vi "Group1Assignment1.vi"() -> ()   [LabVIEW 2020]
doc: "This example performs a serial port write and a serial port read. The parameters set for the serial port must match the parameters of the connected instrument or device. The VISA Configure Serial Port VI sets the configuration parameters. The front panel displays the controls used to configure the basic parameters, such as baud rate, data bits, and parity. The VI passes the VISA resource name to other VIs that perform operations on that VISA resource. The VISA Write function sends a command to the serial device and the VISA Read function returns data based on the command. The VISA Close function then closes the reference to the serial device. It is important to close the reference; otherwise, further communication through that port might not be possible."
uses:
  <vilib>/Utility/file.llb/Write Delimited Spreadsheet (string).vi
  <vilib>/Instr/_visa.llb/VISA Configure Serial Port (Instr).vi
  <vilib>/Utility/file.llb/Read Delimited Spreadsheet (string).vi
  d40ec6dd-3ecf-4240-bb8a-4498ac5227aa.vi
panel:
  out "Table Control":string[][](table)
  out "2D Picture":picture
  in  "error in (no error)":errorcluster
  out "?":u32
  out "Response":string
  in  "VISA resource name":refnum<visa-resource-name>="COM1"
  # "Overview: Demonstrates the use of the VISA functions to send a single command to a serial instrument and read a response.\nRequirements: NI-VISA Driver\nInstructions:\n1. Ensure the resource specified by the VISA resource name is a valid serial device.\n2. Run the VI.\n3. If your instrument recognizes the \"*IDN?\" command, it should return a Response."
  # "Note: For an example of how to perform continuous serial communication in a loop, open the Continuous Serial Write and Read.vi in the same folder as this example."
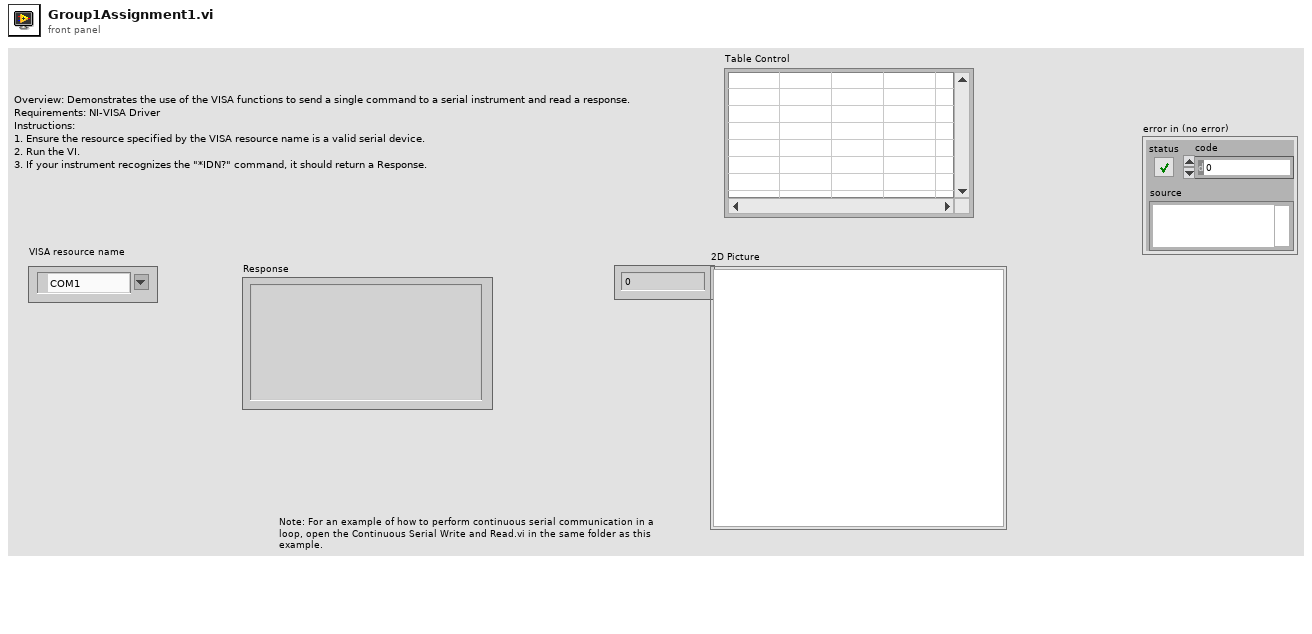
[diagram p1: front panel]
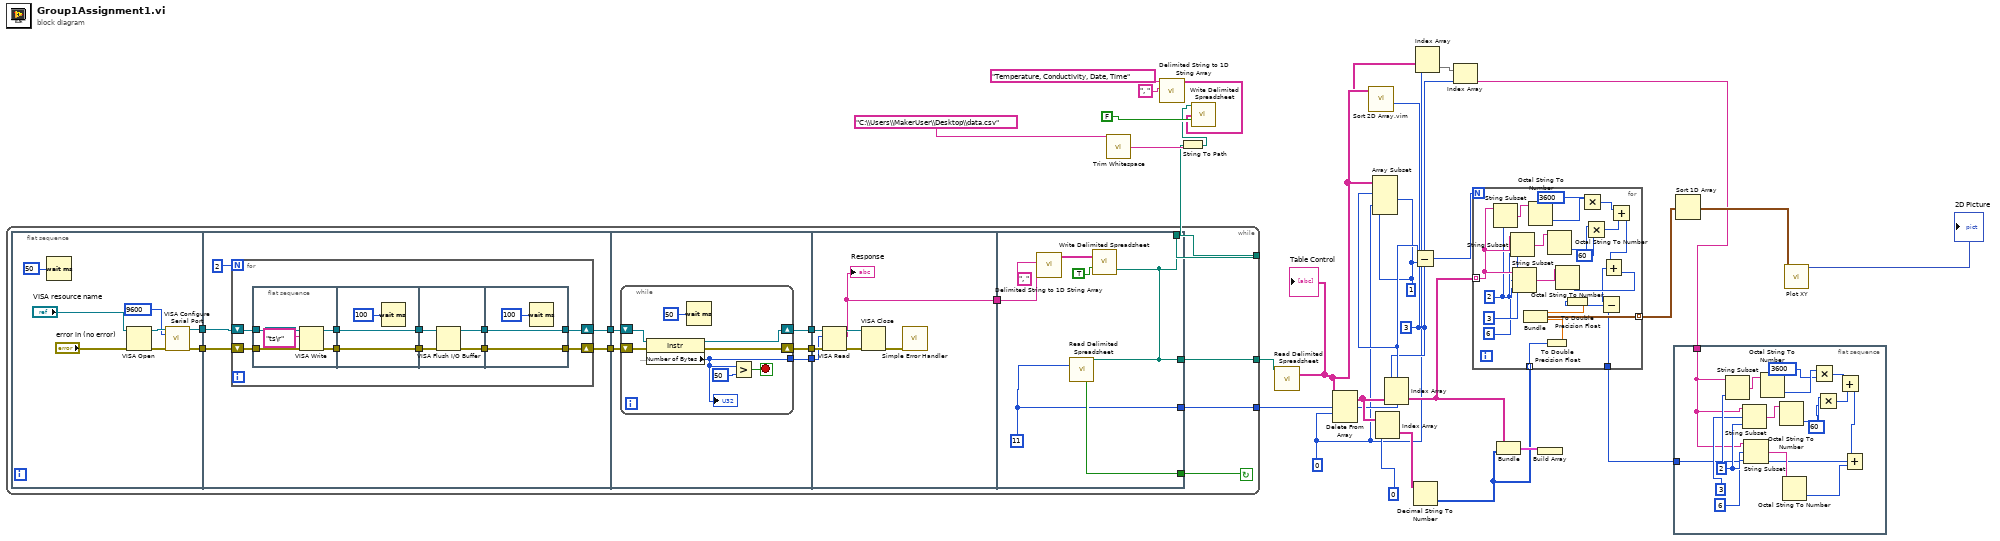
[diagram p0: block diagram]
diagram:
  w5 = 1
  w2 = 3
  w1 = 0
  n1 = call <vilib>:"Trim Whitespace.vi"("string"="C:\\Users\\MakerUser\\Desktop\\data.csv") -> ("trimmed string"=w26:string)  [unwired: 1 in]
  n2 = call <vilib>:"Delimited String to 1D String Array.vi"("delimiter"=", ", "delimited string"="Temperature, Conductivity, Date, Time") -> ("string array"=w23:string[])  [unwired: 9 in]
  n3 = String To Path(string=w26) -> (path=w20:path)
  n4 = while {
    tunnel: w20 -> [w31]
    tunnel: [w29] -> w19
    tunnel: [w28] -> w6
    stop <- w30 continue-if-true
    n5 = flat-sequence {
      tunnel: [w41] -> w39
      tunnel: [w40] -> w38
      tunnel: w39 -> [w52]
      tunnel: w38 -> [w51]
      tunnel: [w49] -> w37
      tunnel: [w48] -> w36
      tunnel: w37 -> [w82]
      tunnel: w36 -> [w81]
      tunnel: [w80] -> w35
      tunnel: [w79] -> w34
      tunnel: [w78] -> w33
      tunnel: w35 -> [w97]
      tunnel: w34 -> [w96]
      tunnel: w33 -> [w95]
      tunnel: [w91] -> w32
      tunnel: w32 -> [w104]
      tunnel: w31 -> [w99]
      tunnel: [w100] -> w30
      tunnel: [w99] -> w29
      tunnel: [w98] -> w28
      frame #0 {
        n6 = Wait (ms)(milliseconds to wait=50) -> ()  [unwired: 1 out]
        n7 = VISA Open(error in (no error)="error in (no error)", VISA resource name="VISA resource name") -> (VISA resource name=w45:refnum<visa-resource-name>, error out=w44:errorcluster)  [unwired: 3 in]
        n8 = call-poly "VISA Configure Serial Port"("VISA resource name"=w45, "baud rate (9600)"=u32 9600, "error in (no error)"=w44) -> ("VISA resource name out"=w41:refnum<visa-resource-name>, "error out"=w40:errorcluster)  [unwired: 6 in, 5 out]
      }
      frame #1 {
        n9 = for {
          N: 2 -> [_]
          shift-right: [w55] -> w49
          shift-left: w52 -> [w54]
          shift-right: [w56] -> w48
          shift-left: w51 -> [w53]
          n10 = flat-sequence {
            tunnel: w54 -> [w66]
            tunnel: w53 -> [w65]
            tunnel: [w64] -> w62
            tunnel: [w63] -> w59
            tunnel: w62 -> [w70]
            tunnel: [w70] -> w61
            tunnel: [w69] -> w60
            tunnel: w59 -> [w69]
            tunnel: w61 -> [w74]
            tunnel: w60 -> [w73]
            tunnel: [w72] -> w58
            tunnel: [w71] -> w57
            tunnel: [w77] -> w55
            tunnel: w58 -> [w77]
            tunnel: [w76] -> w56
            tunnel: w57 -> [w76]
            frame #0 {
              n11 = VISA Write(VISA resource name=w66, write buffer="ts\r", error in (no error)=w65) -> (VISA resource name out=w63:refnum<visa-resource-name>, error out=w64:errorcluster)  [unwired: 1 out]
            }
            frame #1 {
              n12 = Wait (ms)(milliseconds to wait=u32 100) -> ()  [unwired: 1 out]
            }
            frame #2 {
              n13 = VISA Flush I/O Buffer(VISA resource name=w73, error in (no error)=w74) -> (VISA resource name out=w72:refnum<visa-resource-name>, error out=w71:errorcluster)  [unwired: 1 in]
            }
            frame #3 {
              n14 = Wait (ms)(milliseconds to wait=u32 100) -> ()  [unwired: 1 out]
            }
          }
        }
      }
      frame #2 {
        n15 = while {
          tunnel: [w85] -> w78
          shift-right: [w88] -> w79
          shift-left: w81 -> [w83]
          shift-right: [w89] -> w80
          shift-left: w82 -> [w84]
          stop <- w86 stop-if-true
          n16 = property class="Instr"(reference=w84, error in=w83) -> (reference out=w89:refnum<visa-resource-name>, error out=w88:errorcluster, "Serial Settings:Number of Bytes at Serial Port"=w85:u32)
          "?" <- w85
          n17 = Wait (ms)(milliseconds to wait=50) -> ()  [unwired: 1 out]
          n18 = Greater?(x=w85, y=u32 50 ("Serial Settings:Number of Bytes at Serial Port")) -> (0:w86:bool)
        }
      }
      frame #3 {
        n19 = VISA Read(VISA resource name=w97, byte count=w95, error in (no error)=w96) -> (VISA resource name out=w93:refnum<visa-resource-name>, read buffer=w91:string, error out=w92:errorcluster)  [unwired: 1 out]
        "Response" <- w91
        n20 = VISA Close(VISA resource name=w93, error in (no error)=w92) -> (error out=w94:errorcluster)
        n21 = call <vilib>:"Simple Error Handler.vi"("error in (no error)"=w94) -> ()  [unwired: 1 in, 8 out]
      }
      frame #4 {
        w98 = 11
        n22 = call <vilib>:"Delimited String to 1D String Array.vi"("delimiter"=", ", "delimited string"=w104) -> ("string array"=w101:string[])  [unwired: 9 in]
        n23 = call-poly <vilib>:"Read Delimited Spreadsheet.vi"("file path (dialog if empty)"=w99, "number of rows (all:-1)"=w98) -> ("EOF?"=w100:bool)  [unwired: 8 in, 5 out]
        n24 = call-poly <vilib>:"Write Delimited Spreadsheet.vi"("file path (dialog if empty)"=w99, "1D data"=w101, "append to file? (new file:F)"=TRUE) -> ()  [unwired: 11 in, 2 out]
      }
    }
  }
  n25 = call-poly <vilib>:"Write Delimited Spreadsheet.vi"("file path (dialog if empty)"=w20, "1D data"=w23, "append to file? (new file:F)"=FALSE) -> ()  [unwired: 11 in, 2 out]
  n26 = call-poly <vilib>:"Read Delimited Spreadsheet.vi"("file path (dialog if empty)"=w19) -> ("all rows"=w4:string[][])  [unwired: 9 in, 5 out]
  "Table Control" <- w4
  n27 = Delete From Array(array=w4, index (row)=w1) -> (array with subset deleted=w18:string[][])  [unwired: 2 in, 1 out]
  n28 = call "Sort 2D Array.vim"("index"=w2, "2D array"=w4) -> ("sorted 2D array"=w3:string[][])  [unwired: 8 in, 1 out]
  n29 = Array Subset(array=w4, index (row)=w6, length (row)=w5, index (col)=w1, length (col)=w5) -> ()  [unwired: 1 out]
  n30 = Index Array(array=w18, index (col)=0) -> (element=w17:string[])  [unwired: 1 in]
  n31 = Index Array(array=w18, index (col)=w2) -> (element=w13:string[])  [unwired: 1 in]
  n32 = Subtract(x=w6, y=w5) -> (x-y=w15:i32)
  n33 = Decimal String To Number(string=w17) -> (number=w14:i32[])  [unwired: 2 in, 1 out]
  n34 = Index Array(array=w3, index (row)=w1) -> (element=w8:string[])  [unwired: 1 in]
  n35 = Index Array(array=w8, index=w2) -> (element=w7:string)
  n36 = for {
    N: w15 -> [_]
    tunnel: w14 -> [w125] mode=indexing
    tunnel: w13 -> [w122] mode=indexing
    tunnel: [w126] -> w11 mode=indexing
    tunnel: w9 -> [w105]
    w121 = 2
    n37 = String Subset(string=w122, length (rest)=w121) -> (substring=w116:string)  [unwired: 1 in]
    n38 = String Subset(string=w122, offset (0)=3, length (rest)=w121) -> (substring=w118:string)
    n39 = String Subset(string=w122, offset (0)=6, length (rest)=w121) -> (substring=w117:string)
    n40 = Octal String To Number(4:w116) -> (0:w115:u32)  [unwired: 2 in, 1 out]
    n41 = To Double Precision Float(number=w125) -> (double precision float=w124:dbl)
    n42 = Octal String To Number(4:w118) -> (0:w113:u32)  [unwired: 2 in, 1 out]
    n43 = Octal String To Number(4:w117) -> (0:w108:u32)  [unwired: 2 in, 1 out]
    n44 = Multiply(x=w115, y=3600) -> (x*y=w111:u32)
    n45 = Multiply(x=w113, y=60) -> (x*y=w110:u32)
    n46 = Add(x=w111, y=w110) -> (x+y=w109:u32)
    n47 = Add(x=w109, y=w108) -> (x+y=w107:u32)
    n48 = Subtract(x=w107, y=w105) -> (x-y=w106:u32)
    n49 = To Double Precision Float(number=w106) -> (double precision float=w123:dbl)
    n50 = Bundle(w123, w124) -> (w126:cluster{dbl, dbl})  [unwired: 1 in]
  }
  n51 = Bundle("all rows"=w13, w14) -> (w16:cluster{"all rows":string[], i32[]})  [unwired: 1 in]
  n52 = Build Array(w16) -> ()  [unwired: 1 out]
  n53 = flat-sequence {
    tunnel: [w128] -> w9
    tunnel: w7 -> [w127]
    frame #0 {
      w131 = 2
      n54 = String Subset(string=w127, length (rest)=w131) -> (substring=w140:string)  [unwired: 1 in]
      n55 = String Subset(string=w127, offset (0)=3, length (rest)=w131) -> (substring=w142:string)
      n56 = String Subset(string=w127, offset (0)=6, length (rest)=w131) -> (substring=w141:string)
      n57 = Octal String To Number(4:w140) -> (0:w139:u32)  [unwired: 2 in, 1 out]
      n58 = Octal String To Number(4:w142) -> (0:w138:u32)  [unwired: 2 in, 1 out]
      n59 = Octal String To Number(4:w141) -> (0:w135:u32)  [unwired: 2 in, 1 out]
      n60 = Multiply(x=w139, y=3600) -> (x*y=w137:u32)
      n61 = Multiply(x=w138, y=60) -> (x*y=w136:u32)
      n62 = Add(x=w137, y=w136) -> (x+y=w134:u32)
      n63 = Add(x=w134, y=w135) -> (x+y=w128:u32)
    }
  }
  n64 = Sort 1D Array(array=w11) -> (sorted array=w10:cluster{dbl, dbl}[])
  n65 = call <vilib>:"Plot XY.vi"("data"=w10) -> ("new picture"=→"2D Picture":picture)  [unwired: 14 in]
